vi "TPNT_LogType.vi"(8 "error in (no error)":errorcluster, 9 "type in":string, 11 "File":path) -> (0 "error out":errorcluster, 1 "type out":string)   [LabVIEW 2016]
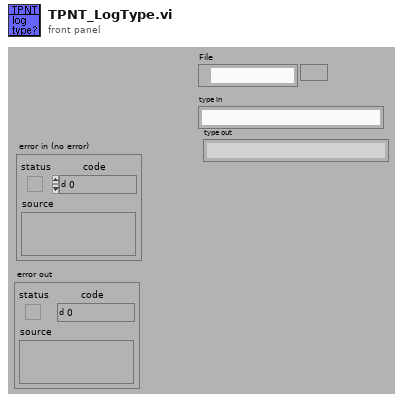
[diagram p1: front panel]
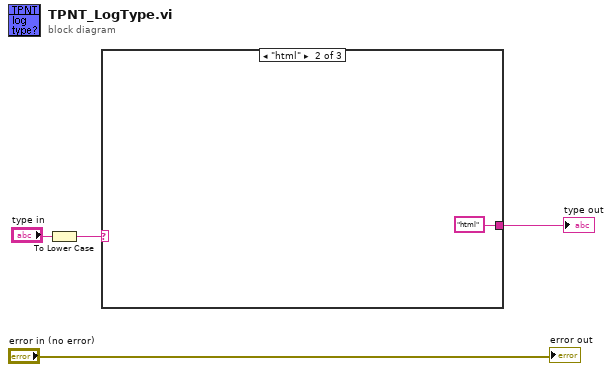
[diagram p0: block diagram]
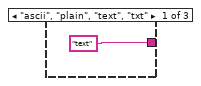
[diagram p2: hidden frame]
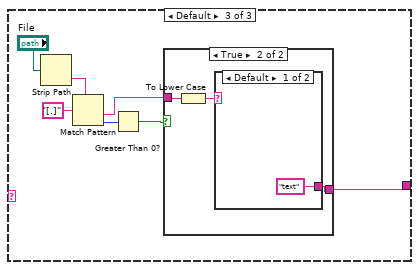
[diagram p3: hidden frame]
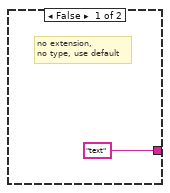
[diagram p4: hidden frame]
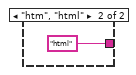
[diagram p5: hidden frame]
diagram:
  n1 = To Lower Case(string="type in") -> (all lower case string=w3:string)
  n2 = case shown="\"html\"" w3 {
    tunnel: ["text" "html" w9] -> w2
    frame "ascii", "plain", "text", "txt" {
    }
    frame "html" {
    }
    frame Default {
      n3 = Strip Path(path="File") -> (name=w12:string)  [unwired: 1 out]
      n4 = Match Pattern(string=w12, regular expression="[.]") -> (after substring=w8:string, offset past match=w11:i32)  [unwired: 3 out]
      n5 = Greater Than 0?(x=w11) -> (x > 0?=w10:bool)
      n6 = case shown="True" w10 {
        tunnel: ["text" w15] -> w9
        tunnel: w8 -> [_ w17]
        frame False {
          # "no extension,\nno type, use default"
        }
        frame True {
          n7 = To Lower Case(string=w17) -> (all lower case string=w16:string)
          n8 = case shown="Default" w16 {
            tunnel: ["text" "html"] -> w15
            frame Default {
            }
            frame "htm", "html" {
            }
          }
        }
      }
    }
  }
  "type out" <- w2
  "error out" <- "error in (no error)"
